vi "Information_Panel.vi"(8 "error in (no error)":errorcluster, 11 "PanelController":refnum<class "MemberPanel.lvclass">) -> (0 "error out":errorcluster, 3 "MemberInfo out":refnum<class "Information.lvclass">)   [LabVIEW 2015, in "Member_Actor.lvlib"]
uses:
  Member_Actor.lvlib
  MemberInfo/Information.lvclass
  MemberPanel/MemberPanel.lvclass
  MemberInfo/Type Definitions/Main Ctl and VI ref.ctl
  MemberInfo/Information.lvclass/Information.ctl
  <vilib>/Utility/error.llb/Error Cluster From Error Code.vi
  <vilib>/ErrorRing/Error Ring.xnode
panel:
  in  "Stop":bool
  in  "组别":enum16{"电控", "机械", "视觉"}(ring)
  in  "操作资料":bool caption="修改信息"
  in  "部门":string
  in  "点击上传照片":bool
  out "照片":picture
  in  "学号":string
  in  "学院":string
  in  "QQ":string
  in  "电话":string
  in  "邮箱":string
  in  "性别":enum16{"男", "女"}(ring)
  in  "年级":string
  in  "姓名":string
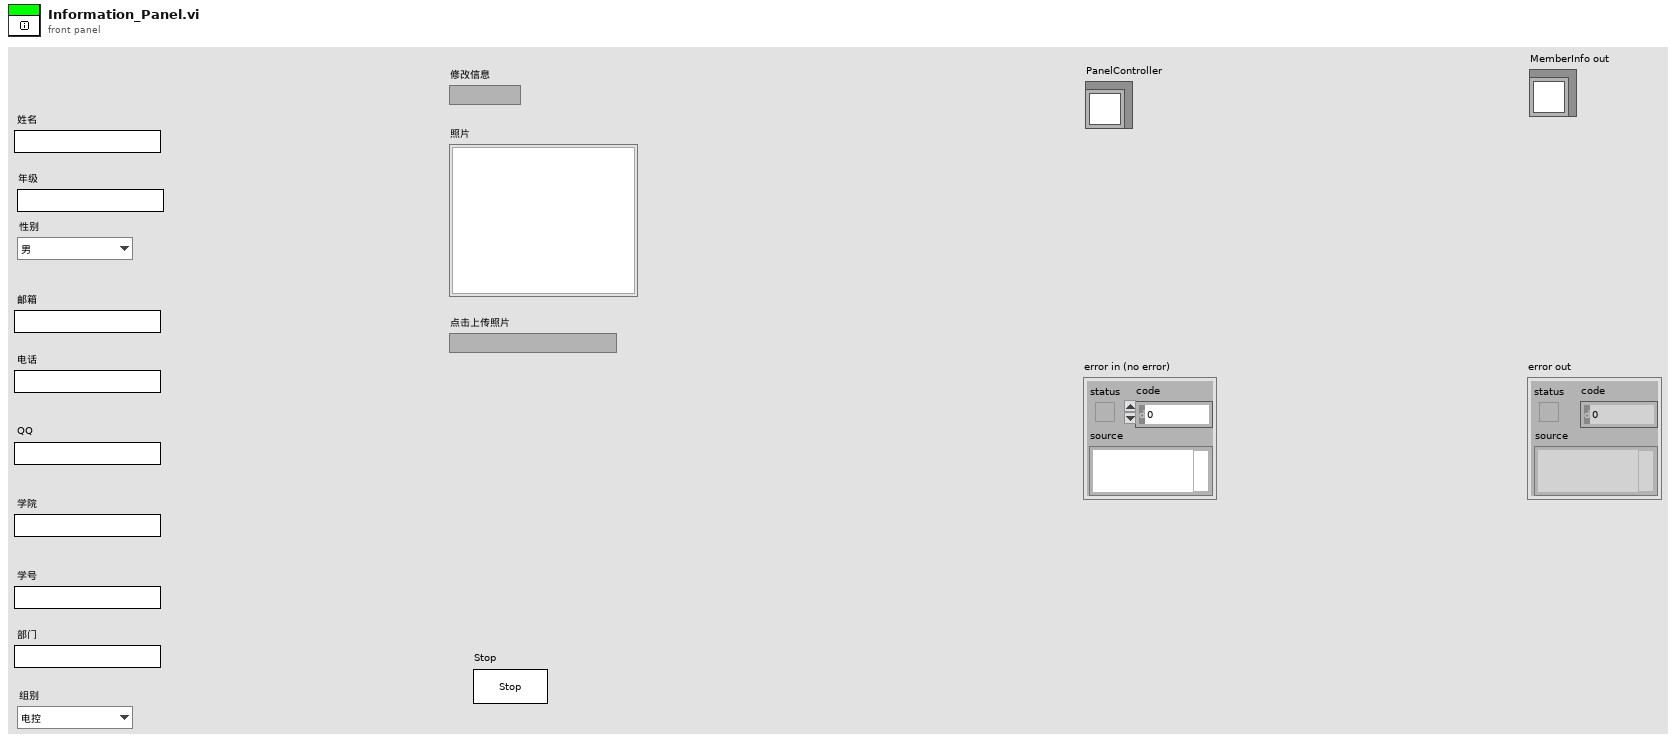
[diagram p1: front panel]
types:
  T1 = typedef "Member_Actor.lvlib/Information.lvclass/Main Ctl and VI ref.ctl" = cluster{"姓名":refnum<vi>, "年级":refnum<vi>, "学号":refnum<vi>, "照片":refnum<vi>, "性别":refnum<vi>, "邮箱":refnum<vi>, "电话":refnum<vi>, "QQ":refnum<vi>, "学院":refnum<vi>, "点击上传照片":refnum<vi>, "操作资料":refnum<vi>, "部门":refnum<vi>, "组别":refnum<vi>}
  T2 = enum32{"Invalid", "Standard", "Closed", "Hidden", "Minimized", "Maximized"}
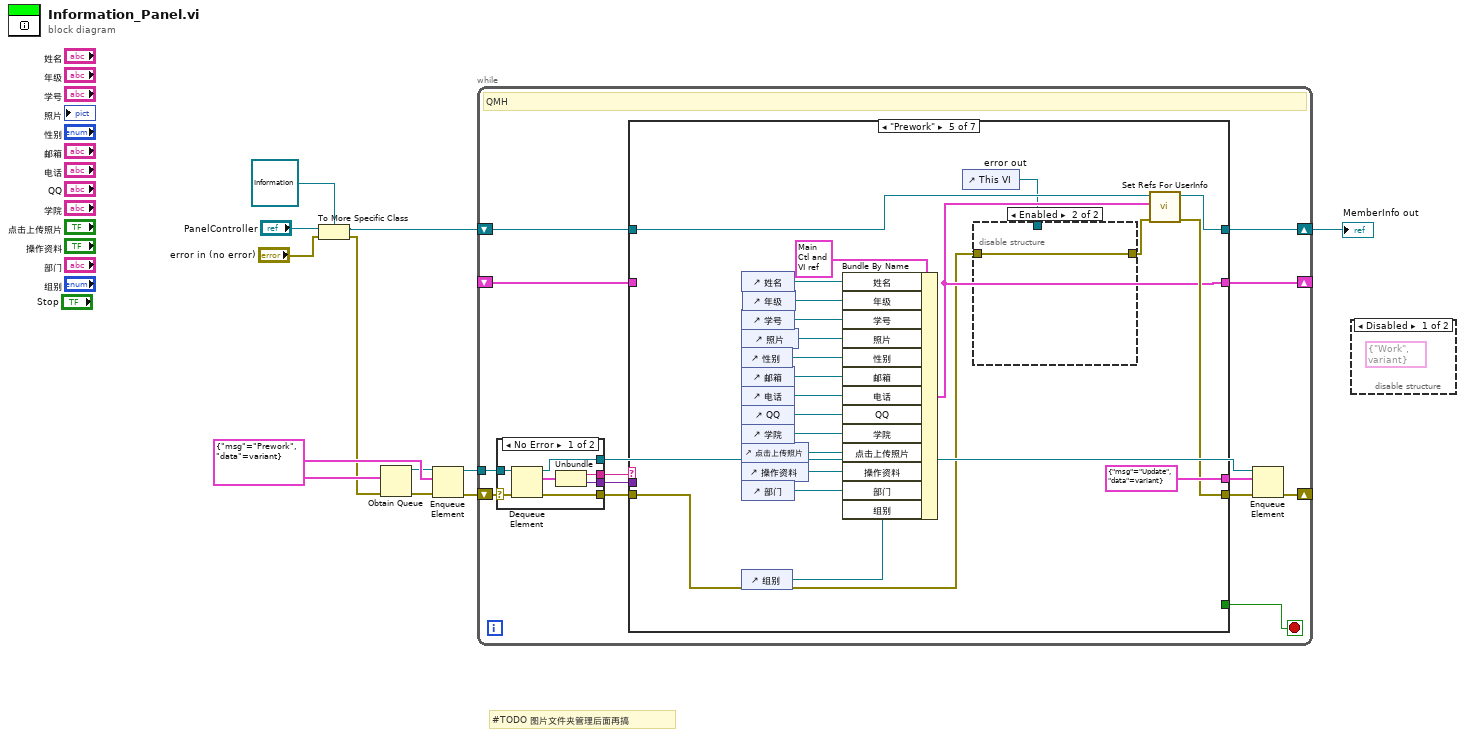
[diagram p0: block diagram]
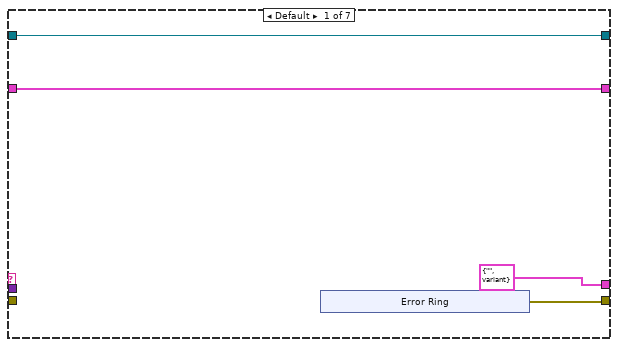
[diagram p3: hidden frame]
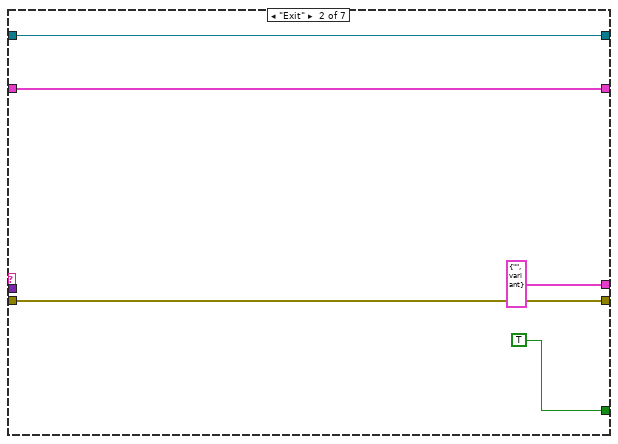
[diagram p4: hidden frame]
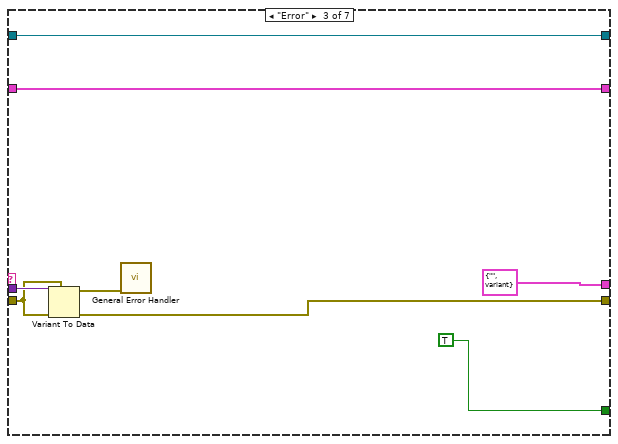
[diagram p5: hidden frame]
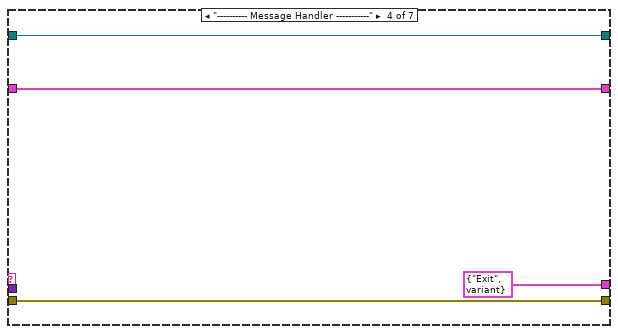
[diagram p6: hidden frame]
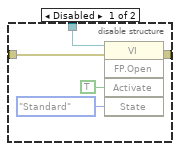
[diagram p7: hidden frame]
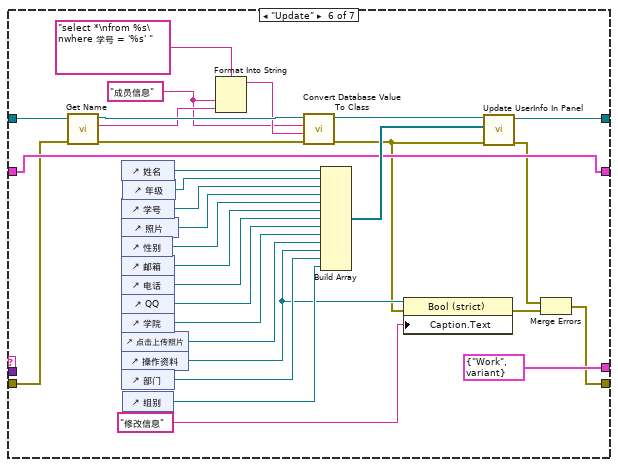
[diagram p8: hidden frame]
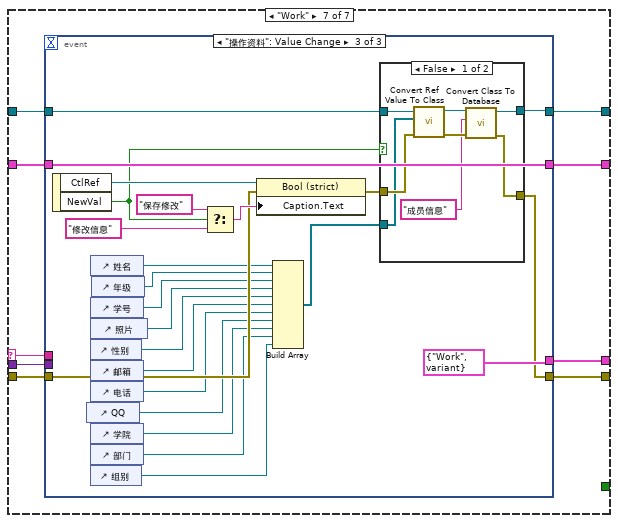
[diagram p9: hidden frame]
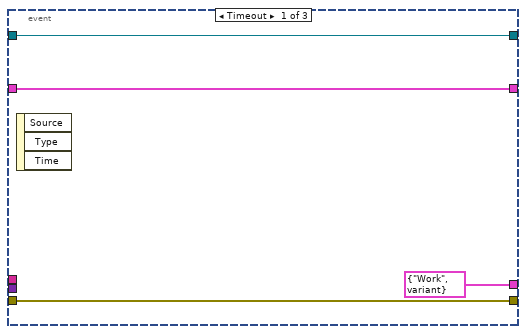
[diagram p10: hidden frame]
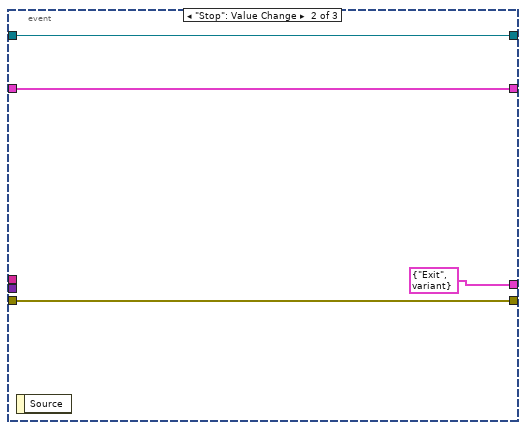
[diagram p11: hidden frame]
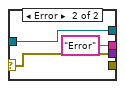
[diagram p13: hidden frame]
diagram:
  w9 = cluster{"msg":string, "data":variant} {"msg"="Prework", "data"=variant}
  # "#TODO 图片文件夹管理后面再搞"
  n1 = To More Specific Class(target class=refnum<class "Information.lvclass"> refnum ("MemberInfo in"), reference="PanelController", error in="error in (no error)") -> (specific class reference=w3:refnum<class "Information.lvclass">, error out=w1:errorcluster)
  n2 = Obtain Queue(element data type=w9, error in (no error)=w1) -> (queue out=w7:refnum<queue>, error out=w8:errorcluster)  [unwired: 3 in, 1 out]
  n3 = Enqueue Element(queue=w7, element=w9, error in (no error)=w8) -> (queue out=w10:refnum<queue>, error out=w11:errorcluster)  [unwired: 1 in, 1 out]
  n4 = while {
    tunnel: w10 -> [w24]
    shift-right: [w19] -> _
    shift-left: w11 -> [w25]
    shift-right: [w14] -> w6
    shift-left: w3 -> [w15]
    shift-right: [w13] -> _
    shift-left: _ -> [w12]
    stop <- w16 stop-if-true
    # "QMH"
    n5 = case shown="No Error" w25 {
      selector: w25 -> [w167 w171]
      tunnel: w24 -> [w168 w169]
      tunnel: [w166 _] -> w23
      tunnel: [w164 "Error" ("msg")] -> w22
      tunnel: [w163 w171] -> w21
      tunnel: [w162 w169] -> w18
      frame No Error {
        n6 = Dequeue Element(queue=w168, error in (no error)=w167) -> (queue out=w162:refnum<queue>, element=w165:cluster{"msg":string, "data":variant}, error out=w166:errorcluster)  [unwired: 1 in, 1 out]
        n7 = Unbundle(w165) -> ("msg"=w164:string, "data"=w163:variant)
      }
      frame Error {
      }
    }
    n8 = case shown="\"Prework\"" w22 {
      selector: w22 -> [_ _ _ _ _ _ w117]
      tunnel: w23 -> [_ w39 w46 w51 w54 w85 w119]
      tunnel: w21 -> [_ _ w47 _ _ _ w118]
      tunnel: [w29 w39 w44 w51 w57 w90 w116] -> w20
      tunnel: [cluster{"msg":string, "data":variant} {"msg"="", "data"=variant} cluster{"msg":string, "data":variant} {"msg"="", "data"=variant} cluster{"msg":string, "data":variant} {"msg"="", "data"=variant} cluster{"msg":string, "data":variant} {"msg"="Exit", "data"=variant} cluster{"msg":string, "data":variant} {"msg"="Update", "data"=variant} cluster{"msg":string, "data":variant} {"msg"="Work", "data"=variant} w115] -> w17
      tunnel: [_ TRUE TRUE _ _ _ _] -> w16
      tunnel: w15 -> [w27 w36 w41 w49 w59 w86 w114]
      tunnel: [w27 w36 w41 w49 w58 w96 w113] -> w14
      tunnel: [w26 w35 w40 w48 w56 w95 w111] -> w13
      tunnel: w12 -> [w26 w35 w40 w48 _ w95 w112]
      frame Default {
        n9 = xnode "Error Ring"() -> ("error out"=w29:errorcluster)
      }
      frame "Exit" {
      }
      frame "Error" {
        n10 = Variant To Data(error in=w46, type=w46, Variant=w47) -> (data=w45:errorcluster, error out=w44:errorcluster)
        n11 = call <vilib>:"General Error Handler.vi"("error in (no error)"=w45) -> ()  [unwired: 10 in, 5 out]
      }
      frame "---------- Message Handler -----------" {
      }
      frame "Prework" {
        n12 = control-ref of="姓名"() -> (w71:refnum<vi>)
        n13 = control-ref of="学号"() -> (w70:refnum<vi>)
        n14 = control-ref of="照片"() -> (w69:refnum<vi>)
        n15 = control-ref of="性别"() -> (w68:refnum<vi>)
        n16 = control-ref of="邮箱"() -> (w67:refnum<vi>)
        n17 = control-ref of="电话"() -> (w66:refnum<vi>)
        n18 = control-ref of="QQ"() -> (w65:refnum<vi>)
        n19 = control-ref of="学院"() -> (w64:refnum<vi>)
        n20 = control-ref of="点击上传照片"() -> (w63:refnum<vi>)
        n21 = control-ref of="操作资料"() -> (w62:refnum<vi>)
        n22 = control-ref of="部门"() -> (w61:refnum<vi>)
        n23 = control-ref of="组别"() -> (w60:refnum<vi>)
        n24 = control-ref of="年级"() -> (w52:refnum<vi>)
        n25 = Bundle By Name(cluster=T1 {"姓名"=refnum, "年级"=refnum, "学号"=refnum, "照片"=refnum, "性别"=refnum, "邮箱"=refnum, "电话"=refnum, "QQ"=refnum, "学院"=refnum, "点击上传照片"=refnum, "操作资料"=refnum, "部门"=refnum, "组别"=refnum} ("Refs"), "姓名"=w71, "年级"=w52, "学号"=w70, "照片"=w69, "性别"=w68, "邮箱"=w67, "电话"=w66, "QQ"=w65, "学院"=w64, "点击上传照片"=w63, "操作资料"=w62, "部门"=w61, "组别"=w60) -> (w56:T1)
        n26 = control-ref of="This VI"() -> (w55:refnum<vi>)
        n27 = disable-structure shown="Enabled" {
          disable-tunnel: w55 -> [w78 _]
          disable-tunnel: w54 -> [w77 w79]
          disable-tunnel: [w76 w79] -> w53
          frame Disabled {
            n28 = invoke class="VI" method="FP.Open"(reference=w78, error in=w77, "Activate"=TRUE ("Activate?"), "State"=T2."Standard") -> (error out=w76:errorcluster)  [unwired: 1 in, 4 out]
          }
          frame Enabled {
          }
        }
        n29 = call "Set Refs For UserInfo.vi"("error in (no error)"=w53, "Refs"=w56, "MemberInfo in"=w59) -> ("error out"=w57:errorcluster, "MemberInfo out"=w58:refnum<class "Information.lvclass">)  [unwired: 7 in]
      }
      frame "Update" {
        w80 = "成员信息" ("input 1")
        n30 = call "Get Name.vi"("error in (no error)"=w85, "MemberInfo in"=w86) -> ("error out"=w83:errorcluster, "学号(\"\")"=w82:string, "MemberInfo out"=w84:refnum<class "Information.lvclass">)  [unwired: 7 in]
        n31 = control-ref of="姓名"() -> (w100:refnum<vi>)
        n32 = control-ref of="学号"() -> (w102:refnum<vi>)
        n33 = control-ref of="照片"() -> (w103:refnum<vi>)
        n34 = control-ref of="性别"() -> (w104:refnum<vi>)
        n35 = control-ref of="邮箱"() -> (w105:refnum<vi>)
        n36 = control-ref of="电话"() -> (w106:refnum<vi>)
        n37 = control-ref of="QQ"() -> (w107:refnum<vi>)
        n38 = control-ref of="学院"() -> (w108:refnum<vi>)
        n39 = control-ref of="点击上传照片"() -> (w109:refnum<vi>)
        n40 = control-ref of="操作资料"() -> (w94:refnum<vi>)
        n41 = control-ref of="部门"() -> (w99:refnum<vi>)
        n42 = control-ref of="年级"() -> (w101:refnum<vi>)
        n43 = control-ref of="组别"() -> (w98:refnum<vi>)
        n44 = Format Into String(format string="select *\nfrom %s\nwhere 学号 = '%s' ", w80, w82) -> (resulting string=w81:string)  [unwired: 2 in, 1 out]
        n45 = call "Convert Database Value To Class.vi"("error in (no error)"=w83, "SQL query"=w81, "Table"=w80, "MemberInfo in"=w84) -> ("error out"=w89:errorcluster, "MemberInfo out"=w88:refnum<class "Information.lvclass">)  [unwired: 6 in]
        n46 = Build Array(w100, w101, w102, w103, w104, w105, w106, w107, w108, w109, w94, w99, w98) -> (w97:refnum<vi>[])
        n47 = property class="Bool (strict)"(reference=w94, error in=w89, "Caption.Text"="修改信息") -> (error out=w92:errorcluster)  [unwired: 1 out]
        n48 = call "Update UserInfo In Panel.vi"("error in (no error)"=w89, "UI Ref"=w97, "MemberInfo in"=w88) -> ("error out"=w91:errorcluster, "MemberInfo out"=w96:refnum<class "Information.lvclass">)  [unwired: 6 in, 1 out]
        n49 = Merge Errors(w91, w92) -> (w90:errorcluster)
      }
      frame "Work" {
        n50 = event shown="[2] \"操作资料\": Value Change" {
          selector: _ -> [_ _ _]
          dyn-events: _ -> [_ _ _]
          timeout: _ -> [_ _ _]
          tunnel: w119 -> [w123 w127 w146]
          tunnel: w118 -> [_ _ _]
          tunnel: w117 -> [_ _ _]
          tunnel: [w123 w127 w129] -> w116
          tunnel: [cluster{"msg":string, "data":variant} {"msg"="Work", "data"=variant} cluster{"msg":string, "data":variant} {"msg"="Exit", "data"=variant} cluster{"msg":string, "data":variant} {"msg"="Work", "data"=variant}] -> w115
          tunnel: w114 -> [w121 w125 w143]
          tunnel: [w121 w125 w128] -> w113
          tunnel: w112 -> [w120 w124 w151]
          tunnel: [w120 w124 w151] -> w111
          event Timeout {
            n51 = event-data() -> ()  [unwired: 1 in, 3 out]
          }
          event "Stop": Value Change {
            n52 = event-data() -> ()  [unwired: 1 in, 1 out]
          }
          event "操作资料": Value Change {
            n53 = event-data() -> ("CtlRef"=w148:refnum<vi>, "NewVal"=w144:bool)  [unwired: 1 in]
            n54 = control-ref of="QQ"() -> (w135:refnum<vi>)
            n55 = control-ref of="姓名"() -> (w142:refnum<vi>)
            n56 = control-ref of="学号"() -> (w140:refnum<vi>)
            n57 = control-ref of="照片"() -> (w139:refnum<vi>)
            n58 = control-ref of="性别"() -> (w138:refnum<vi>)
            n59 = control-ref of="邮箱"() -> (w137:refnum<vi>)
            n60 = control-ref of="电话"() -> (w136:refnum<vi>)
            n61 = control-ref of="学院"() -> (w134:refnum<vi>)
            n62 = control-ref of="部门"() -> (w133:refnum<vi>)
            n63 = control-ref of="组别"() -> (w132:refnum<vi>)
            n64 = control-ref of="年级"() -> (w141:refnum<vi>)
            n65 = Select(t="保存修改", s=w144, f="修改信息") -> (s? t:f=w147:string)
            n66 = property class="Bool (strict)"(reference=w148, error in=w146, "Caption.Text"=w147) -> (error out=w130:errorcluster)  [unwired: 1 out]
            n67 = Build Array(w142, w141, w140, w139, w138, w137, w136, w135, w134, w133, w132) -> (w131:refnum<vi>[])
            n68 = case shown="False" w144 {
              tunnel: w143 -> [w159 w161]
              tunnel: w131 -> [w157 _]
              tunnel: w130 -> [w158 w160]
              tunnel: [w153 w160] -> w129
              tunnel: [w154 w161] -> w128
              frame False {
                n69 = call "Convert Ref Value To Class.vi"("error in (no error)"=w158, "Main Ctls and VI Refs"=w157, "MemberInfo in"=w159) -> ("error out"=w155:errorcluster, "MemberInfo out"=w156:refnum<class "Information.lvclass">)  [unwired: 7 in]
                n70 = call "Convert Class To Database.vi"("error in (no error)"=w155, "table"="成员信息" ("input 1"), "MemberInfo in"=w156) -> ("error out"=w153:errorcluster, "MemberInfo out"=w154:refnum<class "Information.lvclass">)  [unwired: 6 in, 1 out]
              }
              frame True {
              }
            }
          }
        }
      }
    }
    n71 = Enqueue Element(queue=w18, element=w17, error in (no error)=w20) -> (error out=w19:errorcluster)  [unwired: 1 in, 2 out]
  }
  "MemberInfo out" <- w6
  n72 = disable-structure shown="Disabled" {
    frame Disabled {
      (unwired) cluster{"msg":string, "data":variant} {"msg"="Work", "data"=variant}
    }
    frame Enabled {
    }
  }
